vi "Read Manifold Hardware Path.vi"(8 "error in":errorcluster, 10 "Port":i32, 11 "Config Manager in":refnum<class "Config Manager Class.lvclass">) -> (0 "error out":errorcluster, 2 "Hardware Path":string, 3 "Config Manager out":refnum<class "Config Manager Class.lvclass">)   [LabVIEW 2011, in "Config Manager Class.lvclass"]
uses:
  Config Manager Class.lvclass
  Config Manager Class.lvclass/Config Manager Class.ctl
  <vilib>/Utility/config.llb/Read Key (String).vi
  <vilib>/Utility/config.llb/NI_LVConfig.lvlib
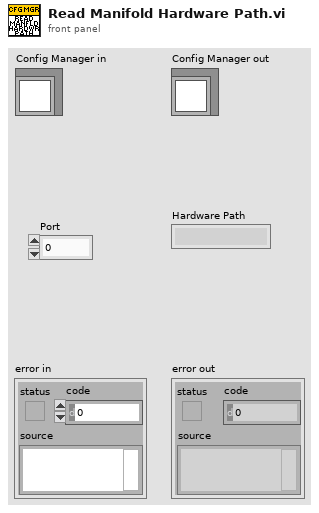
[diagram p1: front panel]
types:
  T1 = typedef "NI_LVConfig.lvlib/Config Data RefNum.ctl" = refnum<k1>
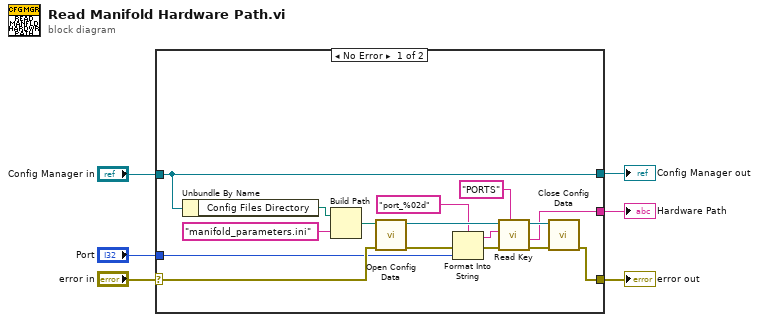
[diagram p0: block diagram]
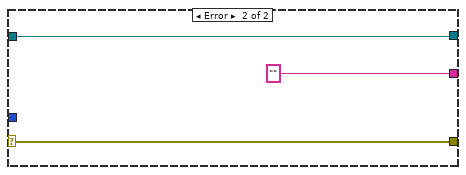
[diagram p2: hidden frame]
diagram:
  n1 = case shown="No Error" "error in" {
    selector: "error in" -> [w22 w25]
    tunnel: [w12 w25] -> w4
    tunnel: [w10 w24] -> w2
    tunnel: "Config Manager in" -> [w10 w24]
    tunnel: "Port" -> [w11 _]
    tunnel: [w7 "" ("value")] -> w1
    frame No Error {
      n2 = Unbundle By Name(w10) -> ("Config Files Directory"=w9:path)
      n3 = Build Path(base path=w9, name or relative path="manifold_parameters.ini") -> (appended path=w8:path)
      n4 = call <vilib>:"Open Config Data.vi"("error in (no error)"=w22, "configuration file path"=w8) -> ("error out"=w18:errorcluster, "refnum"=w19:T1)  [unwired: 7 in, 1 out]
      n5 = Format Into String(format string="port_%02d", error in=w18, w11) -> (resulting string=w16:string, error out=w17:errorcluster)  [unwired: 1 in]
      n6 = call-poly <vilib>:"Read Key.vi"("section"="PORTS", "error in (no error)"=w17, "key"=w16, "refnum"=w19) -> ("error out"=w20:errorcluster, "value"=w7:string, "refnum out"=w21:T1)  [unwired: 4 in, 1 out]
      n7 = call <vilib>:"Close Config Data.vi"("error in (no error)"=w20, "refnum"=w21) -> ("error out"=w12:errorcluster)  [unwired: 8 in, 1 out]
    }
    frame Error {
    }
  }
  "error out" <- w4
  "Config Manager out" <- w2
  "Hardware Path" <- w1
